vi "Enable Output Two Channel.vi"(8 "error in (no error)":errorcluster, 10 "Enable Output (T: Enable)":bool[](array[boolean])=[TRUE, TRUE], 11 "VISA resource name":refnum<visa-resource-name>) -> (0 "error out":errorcluster, 3 "VISA resource name out":refnum<visa-resource-name>)   [LabVIEW 2017, in "Siglent SDG 1000 5000 800 Series.lvlib"]
doc: "Enables or disables the output of the selected channel."
uses:
  <instrlib>/Siglent SDG 1000 5000 800 Series/Siglent SDG 1000 5000 800 Series.lvlib
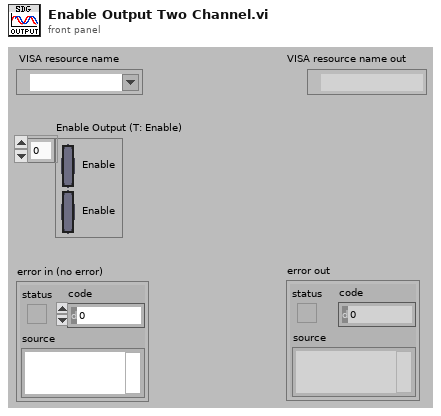
[diagram p1: front panel]
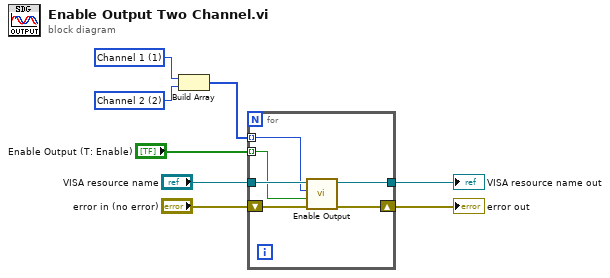
[diagram p0: block diagram]
diagram:
  w8 = 2 items=["Channel 1"=1, "Channel 2"=2] ("Channel (1:Channel 1)")
  w7 = 1 items=["Channel 1"=1, "Channel 2"=2] ("Channel (1:Channel 1)")
  n1 = Build Array(w7, w8) -> (w2:i32[])
  n2 = for {
    tunnel: "VISA resource name" -> [w14]
    tunnel: [w13] -> w5
    shift-right: [w12] -> w4
    shift-left: "error in (no error)" -> [w11]
    tunnel: w2 -> [w10] mode=indexing
    tunnel: "Enable Output (T: Enable)" -> [w9] mode=indexing
    n3 = call <instrlib>:"Enable Output.vi"("error in (no error)"=w11, "Enable Output (T: Enable)"=w9, "Channel (1:Channel 1)"=w10, "VISA resource name"=w14) -> ("error out"=w12:errorcluster, "VISA resource name out"=w13:refnum<visa-resource-name>)  [unwired: 6 in]
  }
  "error out" <- w4
  "VISA resource name out" <- w5
